vi "ReallyComplicatedSonar (SubVI).vi"(11 "Activate Shoot":bool) -> ()   [LabVIEW 2017]
uses:
  <vilib>/Rock Robotics/WPI/Solenoid/WPI_SolenoidValue.ctl
  <vilib>/Rock Robotics/WPI/Utilities/WPI_GetSetVariantRefNum.vi
  <vilib>/Rock Robotics/WPI/RobotDrive/WPI_RobotDriveArcadeDrive_Standard(NoSaturation).vi
  <vilib>/Rock Robotics/WPI/Solenoid/WPI_SolenoidSetEnum.vi
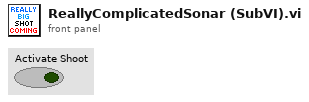
[diagram p1: front panel]
types:
  T1 = typedef "WPI_SolenoidValue.ctl" = enum16{"Off", "On", "Forward", "Reverse"}
  T2 = typedef "WPI_RobotDriveDevRef.ctl" = cluster{"DevStatus":errorcluster, "Motors[]":T3[], "Square Inputs":bool, "Max Output":dbl}
  T3 = typedef "WPI_MotorControlDeviceRef.ctl" = cluster{"DeviceStatus":errorcluster, "Type":T4, "PWM":cluster{"PWM Channel":T5, "DeadBand":T6}, "CAN":cluster{"Device Number":u8, "SetOutput VI Ref":variant, "GetOutput VI Ref":variant, "Enable VI Ref":variant, "Disable VI Ref":variant, "Data":variant}, "Invert":bool, "DIO PWM":cluster{"PWM \"Enable\" Channel":T5, "DIOChannel":T7, "PWM Rate":dbl}}
  T4 = typedef "WPI_MotorControlType.ctl" = enum16{"PWM", "CAN", "DIO PWM"}
  T5 = typedef "FPGA_DIOPWMChannel.ctl" = enum8{"PWM 0", "PWM 1", "PWM 2", "PWM 3", "PWM 4", "PWM 5", "PWM 6", "PWM 7", "PWM 8", "PWM 9", "PWM MXP 0", "PWM MXP 1", "PWM MXP 2", "PWM MXP 3", "PWM MXP 4", "PWM MXP 5", "PWM MXP 6", "PWM MXP 7", "PWM MXP 8", "PWM MXP 9", "Invalid"}
  T6 = typedef "WPI_PWMDeadband.ctl" = cluster{"Name":string, "maxPositivePwm":i32, "minPositivePwm":i32, "centerPwm":i32, "maxNegativePwm":i32, "minNegativePwm":i32, "angularRange":u16}
  T7 = typedef "FPGA_DIOChannel.ctl" = enum8{"DIO 0", "DIO 1", "DIO 2", "DIO 3", "DIO 4", "DIO 5", "DIO 6", "DIO 7", "DIO 8", "DIO 9", "DIO MXP 0", "DIO MXP 1", "DIO MXP 2", "DIO MXP 3", "DIO MXP 4", "DIO MXP 5", "DIO MXP 6", "DIO MXP 7", "DIO MXP 8", "DIO MXP 9", "DIO MXP 10", "DIO MXP 11", "DIO MXP 12", "DIO MXP 13", "DIO MXP 14", "DIO MXP 15", "SPI Port CS1", "SPI Port CS2", "SPI Port CS3", "SPI Port MISO", "SPI Port MOSI", "Invalid"}
  T8 = typedef "DriveMotors.ctl" = cluster{"MotorControlDevRef":T3, "MotorControlDevRef":T3, "MotorControlDevRef":T3, "MotorControlDevRef":T3, "MotorControlDevRef":T3, "MotorControlDevRef":T3}
  T9 = typedef "WPI_SolenoidDevRef.ctl" = cluster{"DevStatus":errorcluster, "Pneumatics Control Module":u8, "Forward Solenoid Channel":T10, "Reverse Solenoid Channel":T10}
  T10 = typedef "WPI_SolenoidChannel.ctl" = enum8{"Solenoid 0", "Solenoid 1", "Solenoid 2", "Solenoid 3", "Solenoid 4", "Solenoid 5", "Solenoid 6", "Solenoid 7", "Invalid"}
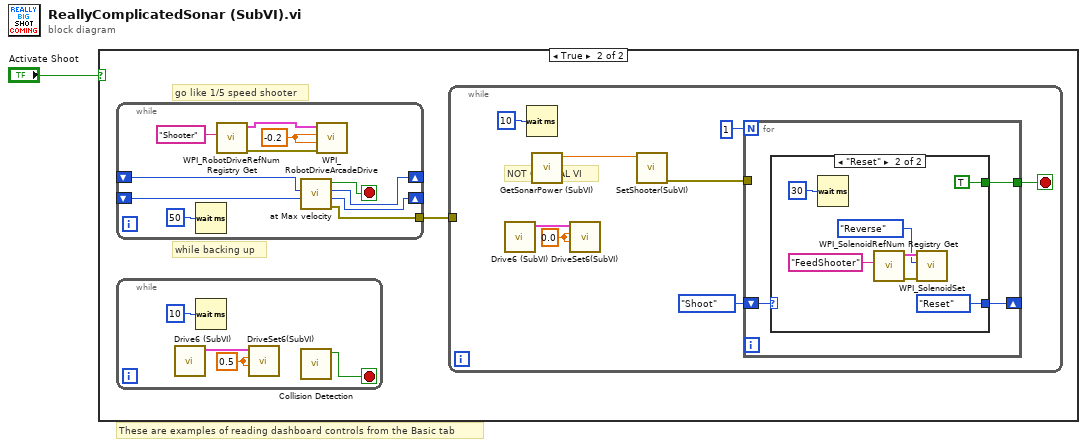
[diagram p0: block diagram]
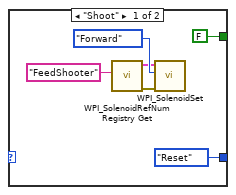
[diagram p3: hidden frame]
diagram:
  # "These are examples of reading dashboard controls from the Basic tab"
  n1 = case shown="True" "Activate Shoot" {
    frame False {
    }
    frame True {
      # "while backing up"
      # "go like 1/5 speed shooter"
      n2 = while {
        shift-right: [w38] -> _
        shift-left: _ -> [w40]
        shift-right: [w36] -> _
        shift-left: _ -> [w39]
        tunnel: [w35] -> w2
        stop <- w37 stop-if-true
        w32 = -0.2 ("Percentage")
        n3 = Wait (ms)(milliseconds to wait=u32 50) -> ()  [unwired: 1 out]
        n4 = call <vilib>:"WPI_RobotDriveRefNum Registry Get.vi"("refnum name"="Shooter") -> ("error out"=w34:errorcluster, "RobotDriveDevRef"=w33:T2)  [unwired: 9 in]
        n5 = call "at Max velocity.vi"("Previous Velocity 2"=w39, "Previous Velocity"=w40) -> ("error out 2"=w35:errorcluster, "New Velocity 2"=w36:i32, "New Velocity"=w38:i32, "Max Velocity"=w37:bool)  [unwired: 6 in]
        n6 = call-poly <vilib>:"WPI_RobotDriveArcadeDrive.vi"("error in (no error)"=w34, "Y axis value"=w32, "X axis value"=w32, "RobotDriveDevRef"=w33) -> ()  [unwired: 5 in, 3 out]
      }
      n7 = while {
        stop <- w30 stop-if-true
        w27 = 0.5 ("Right")
        n8 = call "Drive6 (SubVI).vi"() -> ("DriveControlDevRef"=w28:T8)  [unwired: 11 in]
        n9 = Wait (ms)(milliseconds to wait=u32 10) -> ()  [unwired: 1 out]
        n10 = call "DriveSet6(SubVI).vi"("Left"=w27, "Right"=w27, "output cluster"=w28) -> ()  [unwired: 8 in, 1 out]
        n11 = call "Collision Detection.vi"() -> ("Colision Detected"=w30:bool)  [unwired: 11 in]
      }
      n12 = while {
        tunnel: w2 -> [_]
        stop <- w4 stop-if-true
        w8 = 0.0 ("Right")
        # "NOT OFFICIAL VI"
        n13 = call "Drive6 (SubVI).vi"() -> ("DriveControlDevRef"=w9:T8)  [unwired: 11 in]
        n14 = Wait (ms)(milliseconds to wait=u32 10) -> ()  [unwired: 1 out]
        n15 = call "GetSonarPower (SubVI).vi"() -> ("Value"=w7:dbl)  [unwired: 11 in]
        n16 = call "DriveSet6(SubVI).vi"("Left"=w8, "Right"=w8, "output cluster"=w9) -> ()  [unwired: 8 in, 1 out]
        n17 = call "SetShooter(SubVI).vi"("Velocity"=w7) -> ("error out"=w3:errorcluster)  [unwired: 10 in]
        n18 = for {
          N: 1 -> [_]
          shift-right: [w12] -> _
          shift-left: enum16{"Shoot", "Reset"}."Shoot" -> [w13]
          tunnel: [w11] -> w4
          tunnel: w3 -> [_]
          n19 = case shown="\"Reset\"" w13 {
            tunnel: [enum16{"Shoot", "Reset"}."Reset" enum16{"Shoot", "Reset"}."Reset"] -> w12
            tunnel: [FALSE TRUE] -> w11
            frame "Shoot" {
              n20 = call <vilib>:"WPI_SolenoidRefNum Registry Get.vi"("refnum name"="FeedShooter") -> ("error out"=w16:errorcluster, "SolenoidDevRef"=w17:T9)  [unwired: 9 in]
              n21 = call-poly <vilib>:"WPI_SolenoidSet.vi"("error in (no error)"=w16, "Value"=WPI_SolenoidValue."Forward", "SolenoidDevRef"=w17) -> ()  [unwired: 7 in, 2 out]
            }
            frame "Reset" {
              n22 = Wait (ms)(milliseconds to wait=u32 30) -> ()  [unwired: 1 out]
              n23 = call <vilib>:"WPI_SolenoidRefNum Registry Get.vi"("refnum name"="FeedShooter") -> ("error out"=w25:errorcluster, "SolenoidDevRef"=w26:T9)  [unwired: 9 in]
              n24 = call-poly <vilib>:"WPI_SolenoidSet.vi"("error in (no error)"=w25, "Value"=WPI_SolenoidValue."Reverse", "SolenoidDevRef"=w26) -> ()  [unwired: 7 in, 2 out]
            }
          }
        }
      }
    }
  }
